vi "Acquisition Message Loop.vi"(8 "error in (no error)":errorcluster, 10 "DataQueuesAndNotifier":T1, 11 "Message Queues":T2) -> (0 "error out":errorcluster, 3 "DataQueuesAndNotifier Out":T1)   [LabVIEW 2019, in "Acquisition.lvlib"]
doc: "Message loop for handling messages pertaining to the acquisition of data from the hardware."
uses:
  Acquisition.lvlib
  support/Message Queue/All Message Queues.ctl
  support/Message Queue/Message Cluster.ctl
  DataQueuesAndNotifier.ctl
  Settings/Settings.ctl
  HardwareAdapter/Support/Hardware Configuration.ctl
  HardwareAdapter/Support/Camera Configuration.ctl
  <vilib>/userdefined/High Color/IMAQdx.ctl
  Logging/Logging Configuration.ctl
  controls/UI Configuration.ctl
  controls/CallBack Refs.ctl
  Acquisition State.ctl
  support/Message Queue/Enqueue Message (Single).vi
  <vilib>/Utility/error.llb/Error Cluster From Error Code.vi
  D:/SDK/PMQI-LabViewSamples/Examples/Dependencies/PVCamNET.dll
  E:/DevHardSoftware/MMicroscopy/HardwareAdapter/Lasers/Dependencies/Oxxius_Boxx.dll
  HardwareAdapter/Lasers/Dependencies/Oxxius_Boxx.dll
  <vilib>/ErrorRing/Error Ring.xnode
  support/Message Queue/Message Queue.lvlib
  Settings/Settings.lvlib
  Logging/Logging.lvlib
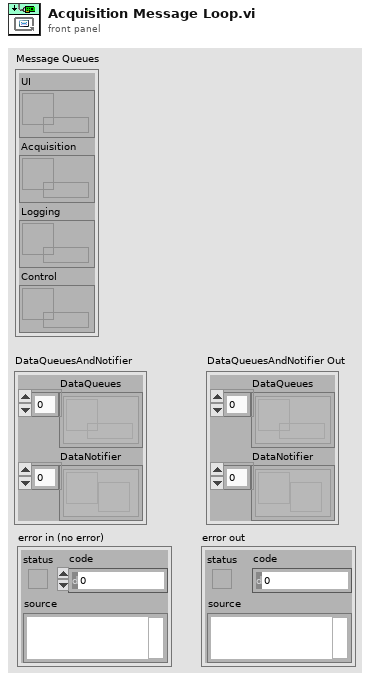
[diagram p1: front panel]
types:
  T1 = typedef "DataQueuesAndNotifier.ctl" = cluster{"DataQueues":refnum<queue>[], "DataNotifier":refnum<notifier>[]}
  T2 = typedef "Message Queue.lvlib/All Message Queues.ctl" = cluster{"UI":refnum<queue>, "Acquisition":refnum<queue>, "Logging":refnum<queue>, "Control":refnum<queue>}
  T3 = typedef "Settings.lvlib/Settings.ctl" = cluster{"Hardware Configuration":T4, "Logging Configuration":T7, "HardWare Status":cluster{"CameraAndStages":T8, "Lasers":cluster{"IsConnected":cluster{"405":bool, "488":bool, "532":bool, "561":bool, "647":bool, "785":bool}, "IsOpened":cluster{"405":bool, "488":bool, "532":bool, "561":bool, "647":bool, "785":bool}}}, "CallBack Ref":T9}
  T4 = typedef "Hardware Configuration.ctl" = cluster{"Camera Configuration":T5, "SimpleCamera Configuration":cluster{"Resource":cluster{"Session Out":T6}}, "Stages Configuration":cluster{"Resource":cluster{"NanoStage Ref":i32, "MicroStage Ref":i32, "TirfLock Ref":i32}, "SettingValues":cluster{"NanoState":cluster{"Time":dbl, "X":dbl, "Y":dbl, "Z":dbl}, "MicroState":cluster{"Time 2":dbl, "Z":dbl}, "TirfLock":cluster{"Time":dbl, "X":dbl, "Y":dbl, "Sum":dbl, "Calbrate":dbl}}}, "Lasers Configuration":cluster{"SettingValues":cluster{"405 Power":sgl, "488 Power":sgl, "532 Power":sgl, "561 Power":sgl, "647 Power":sgl, "785 Power":sgl}, "Resource":cluster{"Library Ref":refnum<k24>, "Lasers Ref":cluster{"405 Ref":refnum<k24>, "488 Ref":refnum<k24>, "532 Ref":refnum<k24>, "561 Ref":refnum<k24>, "647 Ref":refnum<k24>, "785 Ref":refnum<k24>}}}}
  T5 = typedef "Camera Configuration.ctl" = cluster{"Resource":cluster{"CameraRef":refnum<k24>, "LibraryRef":refnum<k24>}, "Setting":cluster{"Expouse":dbl, "Frames":dbl, "Interval":dbl}}
  T6 = typedef "IMAQdx.ctl" = refnum<k21>
  T7 = typedef "Logging.lvlib/Logging Configuration.ctl" = cluster{"Log File Base Path":path, "FilePrefix":string, "TiffFileFullPath":path, "HardWareInfoFileFullPath":path, "NoteFileFullPath":path}
  T8 = typedef "UI Configuration.ctl" = cluster{"Camera":bool, "NanoStage":bool, "MicroStage":bool, "TIRFLock":bool}
  T9 = typedef "CallBack Refs.ctl" = cluster{"event callback refnum":refnum<k27>, "event callback refnum 2":refnum<k27>, "event callback refnum 3":refnum<k27>, "event callback refnum 4":refnum<k27>}
  T10 = typedef "Acquisition.lvlib/Acquisition State.ctl" = enum16{"Idle", "Acquiring", "SequenceAcquire"}
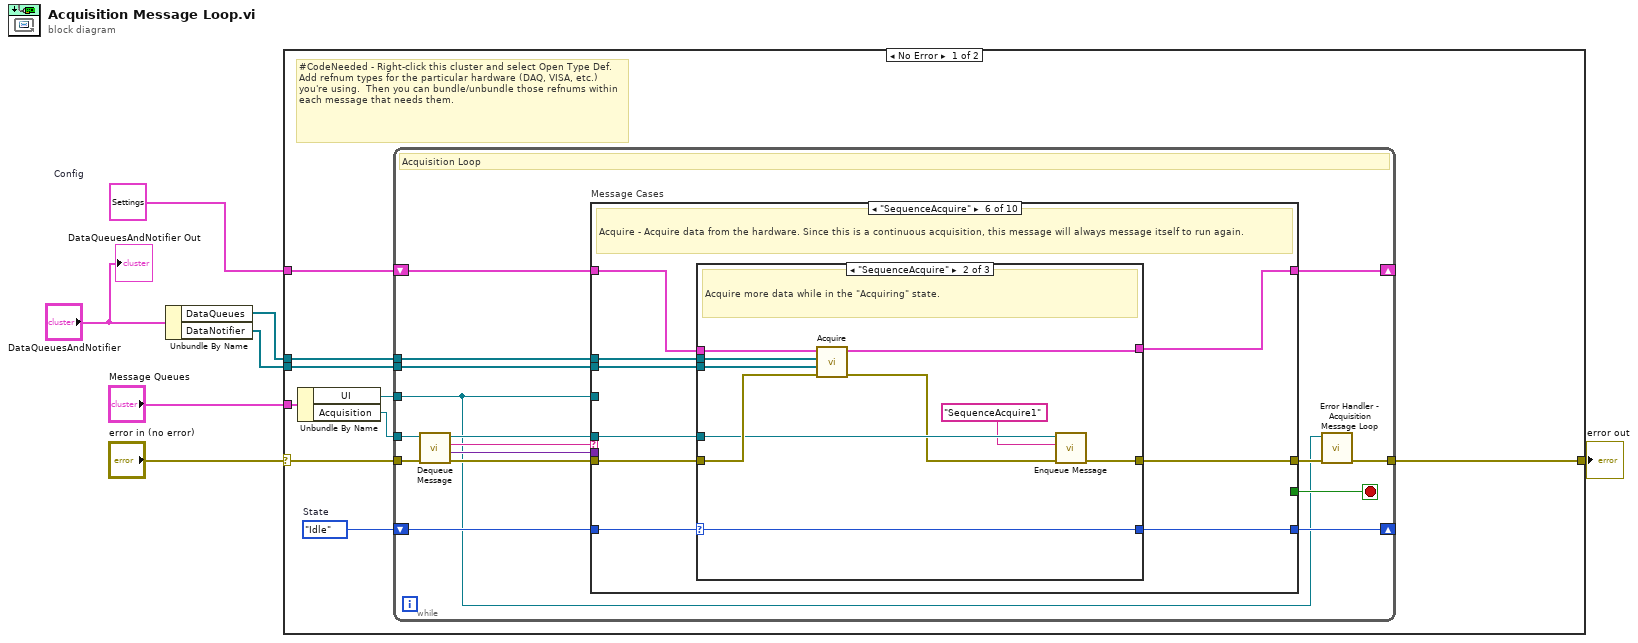
[diagram p0: block diagram]
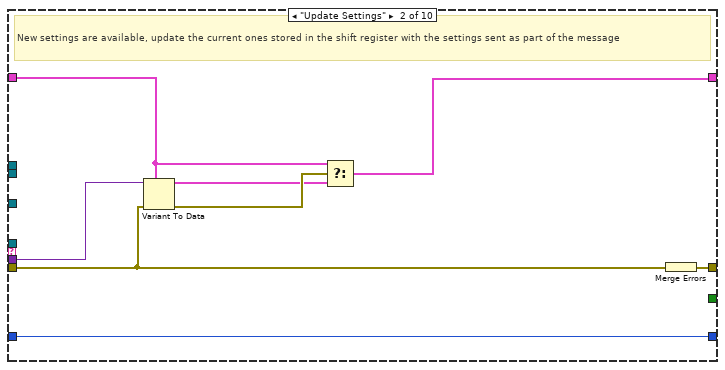
[diagram p3: hidden frame]
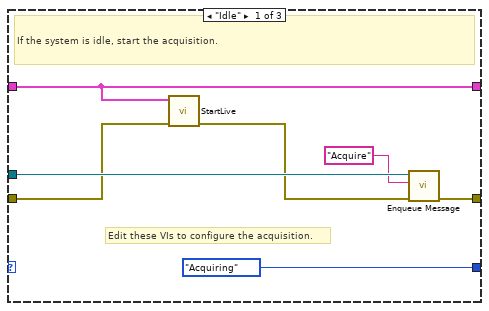
[diagram p5: hidden frame]
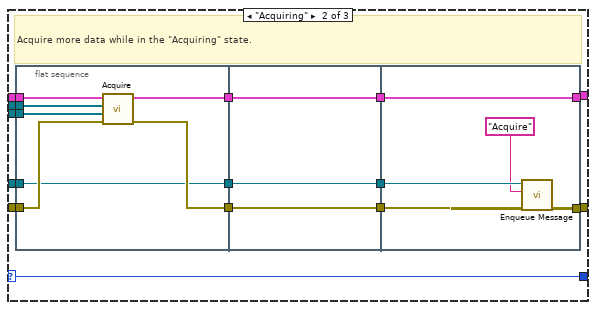
[diagram p9: hidden frame]
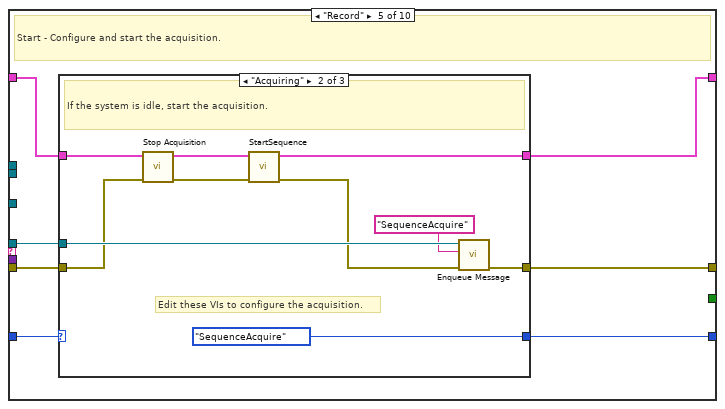
[diagram p10: hidden frame]
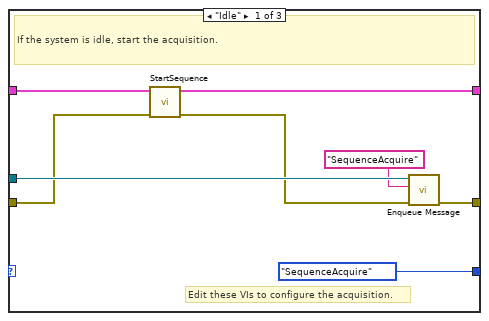
[diagram p11: hidden frame]
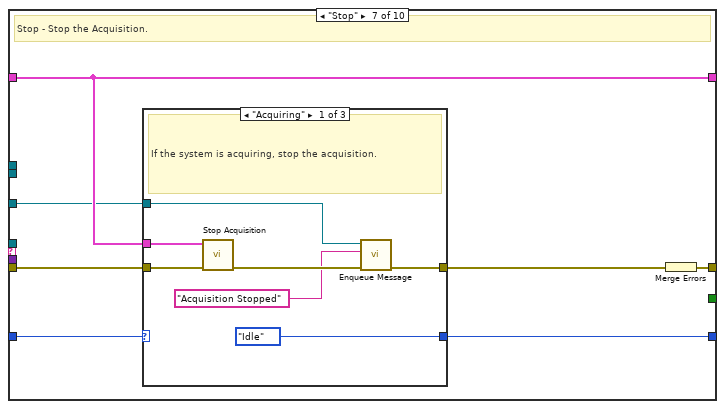
[diagram p15: hidden frame]
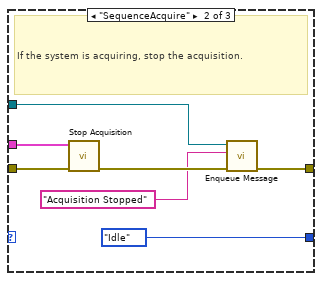
[diagram p16: hidden frame]
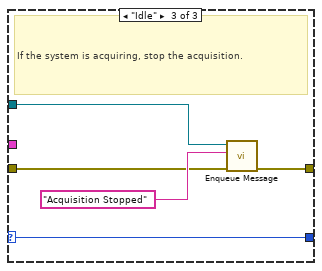
[diagram p17: hidden frame]
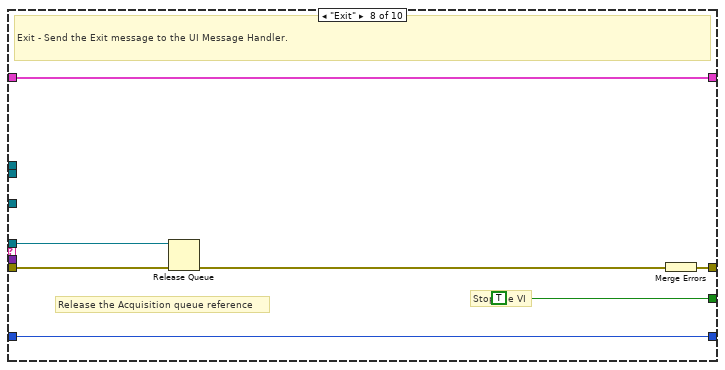
[diagram p18: hidden frame]
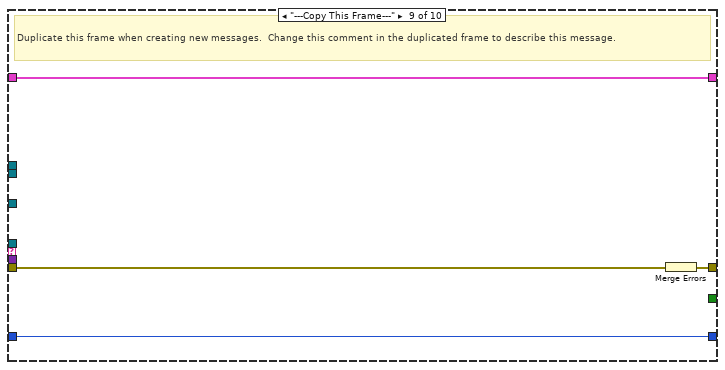
[diagram p19: hidden frame]
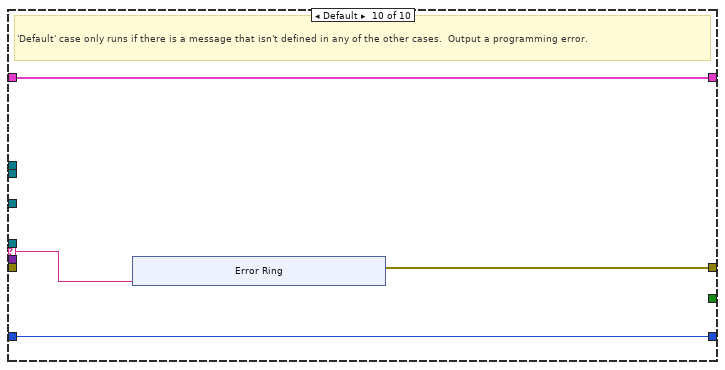
[diagram p20: hidden frame]
diagram:
  w4 = T3 {"Hardware Configuration"={"Camera Configuration"={"Resource"={"CameraRef"=refnum, "LibraryRef"=refnum}, "Setting"={"Expouse"=0.0, "Frames"=0.0, "Interval"=0.0}}, "SimpleCamera Configuration"={"Resource"={"Session Out"=""}}, "Stages Configuration"={"Resource"={"NanoStage Ref"=0, "MicroStage Ref"=0, "TirfLock Ref"=0}, "SettingValues"={"NanoState"={"Time"=0.0, "X"=0.0, "Y"=0.0, "Z"=0.0}, "MicroState"={"Time 2"=0.0, "Z"=0.0}, "TirfLock"={"Time"=0.0, "X"=0.0, "Y"=0.0, "Sum"=0.0, "Calbrate"=0.0}}}, "Lasers Configuration"={"SettingValues"={"405 Power"=0.0, "488 Power"=0.0, "532 Power"=0.0, "561 Power"=0.0, "647 Power"=0.0, "785 Power"=0.0}, "Resource"={"Library Ref"=refnum, "Lasers Ref"={"405 Ref"=refnum, "488 Ref"=refnum, "532 Ref"=refnum, "561 Ref"=refnum, "647 Ref"=refnum, "785 Ref"=refnum}}}}, "Logging Configuration"={"Log File Base Path"=path "", "FilePrefix"="", "TiffFileFullPath"=path "", "HardWareInfoFileFullPath"=path "", "NoteFileFullPath"=path ""}, "HardWare Status"={"CameraAndStages"={"Camera"=FALSE, "NanoStage"=FALSE, "MicroStage"=FALSE, "TIRFLock"=FALSE}, "Lasers"={"IsConnected"={"405"=FALSE, "488"=FALSE, "532"=FALSE, "561"=FALSE, "647"=FALSE, "785"=FALSE}, "IsOpened"={"405"=FALSE, "488"=FALSE, "532"=FALSE, "561"=FALSE, "647"=FALSE, "785"=FALSE}}}, "CallBack Ref"={"event callback refnum"=refnum, "event callback refnum 2"=refnum, "event callback refnum 3"=refnum, "event callback refnum 4"=refnum}}  # Config
  n1 = Unbundle By Name("DataQueuesAndNotifier") -> ("DataQueues"=w3:refnum<queue>[], "DataNotifier"=w2:refnum<notifier>[])
  n2 = case shown="No Error" "error in (no error)" {
    selector: "error in (no error)" -> [w13 w209]
    tunnel: "Message Queues" -> [w16 _]
    tunnel: [w14 w209] -> w6
    tunnel: w3 -> [w10 _]
    tunnel: w2 -> [w9 _]
    tunnel: w4 -> [w8 _]
    frame No Error {
      w11 = Acquisition_State."Idle"  # State
      # "#CodeNeeded - Right-click this cluster and select Open Type Def.  Add refnum types for the particular hardware (DAQ, VISA, etc.) you're using.  Then you can bundle/unbundle those refnums within each message that needs them."
      n3 = Unbundle By Name(w16) -> ("UI"=w12:refnum<queue>, "Acquisition"=w15:refnum<queue>)
      n4 = while {
        tunnel: w15 -> [w25]
        shift-right: [w31] -> _
        shift-left: w8 -> [w32]
        tunnel: w12 -> [w19]
        shift-right: [w23] -> _
        shift-left: w11 -> [w24]
        tunnel: w13 -> [w29]
        tunnel: [w22] -> w14
        tunnel: w10 -> [w18]
        tunnel: w9 -> [w17]
        stop <- w30 stop-if-true
        # "Acquisition Loop"
        n5 = call "Dequeue Message.vi"("error in (no error)"=w29, "Message Queue"=w25) -> ("error out"=w28:errorcluster, "Message Data"=w26:variant, "Message"=w27:string, "dup Message Queue"=w20:refnum<queue>)  [unwired: 6 in]
        n6 = case "Message Cases" shown="\"SequenceAcquire\"" w27 {
          selector: w27 -> [_ _ _ _ _ _ _ _ _ w198]
          tunnel: w20 -> [_ _ w47 w71 w111 w143 _ w191 _ _]
          tunnel: w28 -> [w35 w37 w48 w70 w112 w142 w166 w188 w197 _]
          tunnel: [w35 w43 w50 w72 w114 w144 w167 w192 w195 w199] -> w21
          tunnel: w32 -> [w34 w39 w49 w68 w113 w140 w164 w187 w196 w201]
          tunnel: [w34 w38 w46 w69 w110 w141 w164 w187 w196 w201] -> w31
          tunnel: [_ _ _ _ _ _ _ TRUE _ _] -> w30
          tunnel: w26 -> [_ w42 _ _ _ _ _ _ _ _]
          tunnel: w19 -> [_ _ _ _ _ _ w161 _ _ _]
          tunnel: w24 -> [w33 w36 w44 w66 w108 w138 w163 w190 w194 w200]
          tunnel: [w33 w36 w45 w67 w109 w139 w162 w190 w194 w200] -> w23
          tunnel: w18 -> [_ _ _ w65 _ w137 _ _ _ _]
          tunnel: w17 -> [_ _ _ w64 _ w136 _ _ _ _]
          frame "Initialize" {
            # "Initialize  - Initialize is currently a no-op.  The hardware initialization takes place in the 'Start' message."
          }
          frame "Update Settings" {
            # "New settings are available, update the current ones stored in the shift register with the settings sent as part of the message"
            n7 = Variant To Data(error in=w37, type=w39, Variant=w42) -> (data=w40:T3, error out=w41:errorcluster)
            n8 = Select(t=w39, s=w41, f=w40) -> (s? t:f=w38:T3)
            n9 = Merge Errors(w37) -> (w43:errorcluster)
          }
          frame "Live" {
            # "Start - Configure and start the acquisition."
            n10 = case shown="\"Acquiring\"" w44 {
              selector: w44 -> [_ w58 w61]
              tunnel: [w51 w59 w63] -> w50
              tunnel: w49 -> [w54 w60 w62]
              tunnel: w48 -> [w53 w59 w63]
              tunnel: w47 -> [w57 _ _]
              tunnel: [w54 w60 w62] -> w46
              tunnel: [Acquisition_State."Acquiring" ("Acquisition State") w58 w61] -> w45
              frame "Idle" {
                # "Edit these VIs to configure the acquisition."
                # "If the system is idle, start the acquisition."
                n11 = call "StartLive.vi"("error in (no error)"=w53, "Config In"=w54) -> ("error out"=w52:errorcluster)  [unwired: 8 in, 1 out]
                n12 = call-poly "Enqueue Message.vi"("error in (no error)"=w52, "Message"="Acquire", "Message Queue"=w57) -> ("error out"=w51:errorcluster)  [unwired: 7 in, 1 out]
              }
              frame "Acquiring" {
                # "The system is already acquiring. Ignore the \"Start\" message."
              }
              frame "SequenceAcquire" {
              }
            }
          }
          frame "Acquire" {
            # "Acquire - Acquire data from the hardware. Since this is a continuous acquisition, this message will always message itself to run again."
            n13 = case shown="\"SequenceAcquire\"" w66 {
              selector: w66 -> [w73 w89 w105]
              tunnel: [w74 w83 w107] -> w72
              tunnel: w71 -> [_ w82 _]
              tunnel: w70 -> [w74 w88 w107]
              tunnel: [w75 w84 w106] -> w69
              tunnel: w68 -> [w75 w87 w106]
              tunnel: [w73 w89 w105] -> w67
              tunnel: w65 -> [_ w86 _]
              tunnel: w64 -> [_ w85 _]
              frame "Idle" {
                # "Ignore \"Acquire\" messages when the acquisition is idle."
              }
              frame "Acquiring" {
                # "Acquire more data while in the \"Acquiring\" state."
                n14 = flat-sequence {
                  tunnel: w88 -> [w96]
                  tunnel: w87 -> [w95]
                  tunnel: w86 -> [w94]
                  tunnel: w85 -> [w93]
                  tunnel: [w92] -> w81
                  tunnel: [w91] -> w79
                  tunnel: [w90] -> w77
                  tunnel: w82 -> [w90]
                  tunnel: w81 -> [w99]
                  tunnel: [w99] -> w80
                  tunnel: w79 -> [w98]
                  tunnel: [w98] -> w78
                  tunnel: w77 -> [w97]
                  tunnel: [w97] -> w76
                  tunnel: [w104] -> w84
                  tunnel: w80 -> [w104]
                  tunnel: w78 -> [w103]
                  tunnel: [w102] -> w83
                  tunnel: w76 -> [w101]
                  frame #0 {
                    n15 = call "Acquire.vi"("error in (no error)"=w96, "DataNotifier"=w93, "DataQueues"=w94, "Config In"=w95) -> ("error out"=w91:errorcluster, "Config Out"=w92:T3)  [unwired: 6 in]
                  }
                  frame #1 {
                  }
                  frame #2 {
                    n16 = call-poly "Enqueue Message.vi"("error in (no error)"=w103, "Message"="Acquire", "Message Queue"=w101) -> ("error out"=w102:errorcluster)  [unwired: 7 in, 1 out]
                  }
                }
              }
              frame "SequenceAcquire" {
              }
            }
          }
          frame "Record" {
            # "Start - Configure and start the acquisition."
            n17 = case shown="\"Acquiring\"" w108 {
              selector: w108 -> [_ _ w133]
              tunnel: [w118 w128 w135] -> w114
              tunnel: w113 -> [w115 w125 w134]
              tunnel: w112 -> [w116 w126 w135]
              tunnel: w111 -> [w122 w132 _]
              tunnel: [w117 w127 w134] -> w110
              tunnel: [Acquisition_State."SequenceAcquire" ("Acquisition State") Acquisition_State."SequenceAcquire" ("Acquisition State") w133] -> w109
              frame "Idle" {
                # "Edit these VIs to configure the acquisition."
                # "If the system is idle, start the acquisition."
                n18 = call "StartSequence.vi"("error in (no error)"=w116, "Config In"=w115) -> ("error out"=w119:errorcluster, "Config Out"=w117:T3)  [unwired: 8 in]
                n19 = call-poly "Enqueue Message.vi"("error in (no error)"=w119, "Message"="SequenceAcquire", "Message Queue"=w122) -> ("error out"=w118:errorcluster)  [unwired: 7 in, 1 out]
              }
              frame "Acquiring" {
                # "Edit these VIs to configure the acquisition."
                # "If the system is idle, start the acquisition."
                n20 = call "Stop Acquisition.vi"("error in (no error)"=w126, "Config"=w125) -> ("error out"=w124:errorcluster, "Config Out"=w123:T3)  [unwired: 8 in]
                n21 = call "StartSequence.vi"("error in (no error)"=w124, "Config In"=w123) -> ("error out"=w129:errorcluster, "Config Out"=w127:T3)  [unwired: 8 in]
                n22 = call-poly "Enqueue Message.vi"("error in (no error)"=w129, "Message"="SequenceAcquire", "Message Queue"=w132) -> ("error out"=w128:errorcluster)  [unwired: 7 in, 1 out]
              }
              frame "SequenceAcquire" {
              }
            }
          }
          frame "SequenceAcquire" {
            # "Acquire - Acquire data from the hardware. Since this is a continuous acquisition, this message will always message itself to run again."
            n23 = case shown="\"SequenceAcquire\"" w138 {
              selector: w138 -> [w145 w156 w158]
              tunnel: [w146 w157 w160] -> w144
              tunnel: w143 -> [_ w150 _]
              tunnel: w142 -> [w146 w155 w160]
              tunnel: [w147 w151 w159] -> w141
              tunnel: w140 -> [w147 w154 w159]
              tunnel: [w145 w156 w158] -> w139
              tunnel: w137 -> [_ w153 _]
              tunnel: w136 -> [_ w152 _]
              frame "Idle" {
                # "Ignore \"Acquire\" messages when the acquisition is idle."
              }
              frame "SequenceAcquire" {
                # "Acquire more data while in the \"Acquiring\" state."
                n24 = call "Acquire.vi"("error in (no error)"=w155, "DataNotifier"=w152, "DataQueues"=w153, "Config In"=w154) -> ("error out"=w149:errorcluster, "Config Out"=w151:T3)  [unwired: 6 in]
                n25 = call-poly "Enqueue Message.vi"("error in (no error)"=w149, "Message"="SequenceAcquire1", "Message Queue"=w150) -> ("error out"=w157:errorcluster)  [unwired: 7 in, 1 out]
              }
              frame "Acquiring" {
              }
            }
          }
          frame "Stop" {
            # "Stop - Stop the Acquisition."
            n26 = case shown="\"Acquiring\"" w163 {
              selector: w163 -> [_ _ w182]
              tunnel: w166 -> [w174 w181 w183]
              tunnel: [w171 w178 w186] -> w165
              tunnel: w164 -> [w168 w175 _]
              tunnel: [Acquisition_State."Idle" ("State") Acquisition_State."Idle" ("State") w182] -> w162
              tunnel: w161 -> [w170 w177 w185]
              frame "Acquiring" {
                # "If the system is acquiring, stop the acquisition."
                n27 = call "Stop Acquisition.vi"("error in (no error)"=w174, "Config"=w168) -> ("error out"=w173:errorcluster)  [unwired: 8 in, 1 out]
                n28 = call-poly "Enqueue Message.vi"("error in (no error)"=w173, "Message"="Acquisition Stopped", "Message Queue"=w170) -> ("error out"=w171:errorcluster)  [unwired: 7 in, 1 out]
              }
              frame "SequenceAcquire" {
                # "If the system is acquiring, stop the acquisition."
                n29 = call "Stop Acquisition.vi"("error in (no error)"=w181, "Config"=w175) -> ("error out"=w180:errorcluster)  [unwired: 8 in, 1 out]
                n30 = call-poly "Enqueue Message.vi"("error in (no error)"=w180, "Message"="Acquisition Stopped", "Message Queue"=w177) -> ("error out"=w178:errorcluster)  [unwired: 7 in, 1 out]
              }
              frame "Idle" {
                # "If the system is acquiring, stop the acquisition."
                n31 = call-poly "Enqueue Message.vi"("error in (no error)"=w183, "Message"="Acquisition Stopped", "Message Queue"=w185) -> ("error out"=w186:errorcluster)  [unwired: 7 in, 1 out]
              }
            }
            n32 = Merge Errors(w165) -> (w167:errorcluster)
          }
          frame "Exit" {
            # "Release the Acquisition queue reference"
            # "Stop the VI"
            # "Exit - Send the Exit message to the UI Message Handler."
            n33 = Release Queue(queue=w191, error in (no error)=w188) -> (error out=w189:errorcluster)  [unwired: 1 in, 2 out]
            n34 = Merge Errors(w189) -> (w192:errorcluster)
          }
          frame "---Copy This Frame---" {
            # "Duplicate this frame when creating new messages.  Change this comment in the duplicated frame to describe this message."
            n35 = Merge Errors(w197) -> (w195:errorcluster)
          }
          frame Default {
            # "'Default' case only runs if there is a message that isn't defined in any of the other cases.  Output a programming error."
            n36 = xnode "Error Ring"("parameter 0"=w198) -> ("error out"=w199:errorcluster)
          }
        }
        n37 = call "Error Handler - Acquisition Message Loop.vi"("error in (no error)"=w21, "Message Queue"=w19) -> ("dup error in"=w22:errorcluster)  [unwired: 8 in, 1 out]
      }
    }
    frame Error {
    }
  }
  "error out" <- w6
  "DataQueuesAndNotifier Out" <- "DataQueuesAndNotifier"
